vi "Setup Pressure Sensor Settings.vi"(8 "error in (no error)":errorcluster, 10 "Model in":refnum<class "Model.lvclass">, 11 "Boot Loader in":refnum<class "Boot Loader.lvclass">) -> (0 "error out":errorcluster, 2 "Model out":refnum<class "Model.lvclass">, 3 "Boot Loader out":refnum<class "Boot Loader.lvclass">)   [LabVIEW 2015, in "Boot Loader.lvclass"]
uses:
  Boot Loader.lvclass
  Model/Model.lvclass
  Model/Model.lvclass/Model.ctl
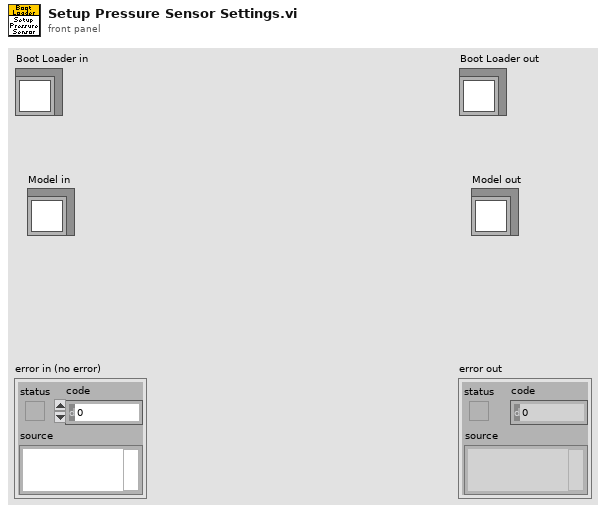
[diagram p1: front panel]
types:
  T1 = typedef "FAMT Typedefs.lvlib/Pressure Sensor Settings.ctl" = cluster{"Read Pressures":bool, "Volts per PSI":dbl, "Offset":dbl}
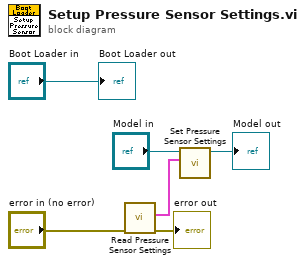
[diagram p0: block diagram]
diagram:
  n1 = call "Read Pressure Sensor Settings.vi"("error in (no error)"="error in (no error)") -> ("error out"=→"error out":errorcluster, "Pressure Sensor Settings"=w1:T1)  [unwired: 8 in, 1 out]
  n2 = call "Set Pressure Sensor Settings.vi"("Pressure Sensor Settings"=w1, "Model in"="Model in") -> ("Model out"=→"Model out":refnum<class "Model.lvclass">)  [unwired: 9 in]
  "Boot Loader out" <- "Boot Loader in"
